vi "Telnet_Open.vi"(8 "Error In":errorcluster caption="Entrée d'erreur", 9 "Timeout(ms)":i32=1000, 10 "RemotePort(23)":u16=23, 11 "HostAddress":string="192.168.1.200") -> (0 "Error Out":errorcluster caption="Sortie d'erreur", 2 "telnet connection":T1, 3 "Status":bool)   [LabVIEW 2013]
uses:
  <vilib>/addons/internet/telnet/telnet.llb/Telnet Session.ctl
  <vilib>/addons/internet/NI_InternetTK_Core_VIs.lvlib
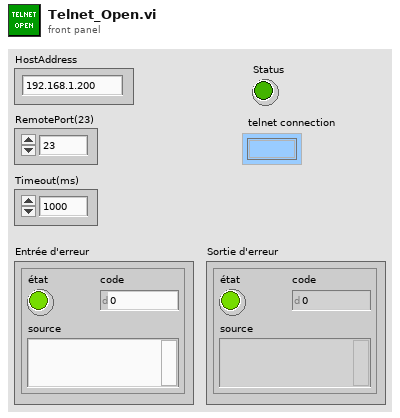
[diagram p1: front panel]
types:
  T1 = typedef "Telnet Session.ctl" = refnum<k1>
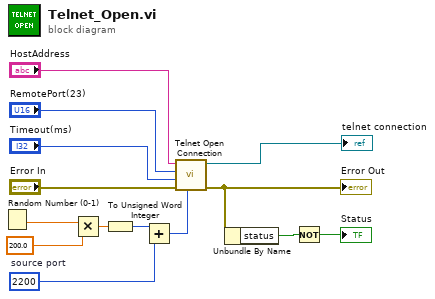
[diagram p0: block diagram]
diagram:
  w7 = u16 2200  # source port
  n1 = Random Number (0-1)() -> (number: 0 to 1=w9:dbl)
  n2 = Multiply(x=w9, y=200.0) -> (x*y=w11:dbl)
  n3 = To Unsigned Word Integer(number=w11) -> (unsigned 16bit integer=w8:u16)
  n4 = Add(x=w8, y=w7) -> (x+y=w6:u16)
  n5 = call <vilib>:"Telnet Open Connection.vi"("local port"=w6, "error in (no error)"="Error In", "timeout ms (60000)"="Timeout(ms)", "remote port (23)"="RemotePort(23)", "address"="HostAddress") -> ("error out"=w3:errorcluster, "telnet connection"=→"telnet connection":T1)  [unwired: 5 in]
  "Error Out" <- w3
  n6 = Unbundle By Name(w3) -> ("status"=w2:bool)
  n7 = Not(x=w2) -> (.not. x?=→"Status":bool)
